vi "Write Duration.vi"(8 "error in (no error)":errorcluster, 10 "Duration":u32 caption="ms" step=1 format="%.0g", 11 "TimedDirector in":refnum<class "TimedDirector.lvclass">) -> (0 "error out":errorcluster, 3 "TimedDirector out":refnum<class "TimedDirector.lvclass">)   [LabVIEW 2023, in "HAF.lvlib" / "TimedDirector.lvclass"]
uses:
  TimedDirector.lvclass
  TimedDirector.lvclass/TimedDirector.ctl
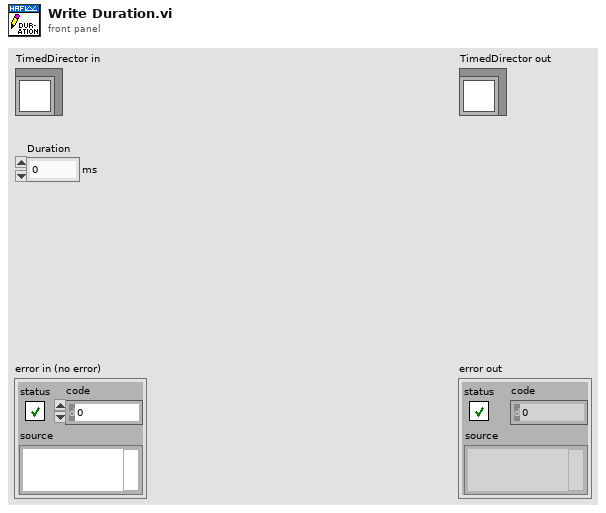
[diagram p1: front panel]
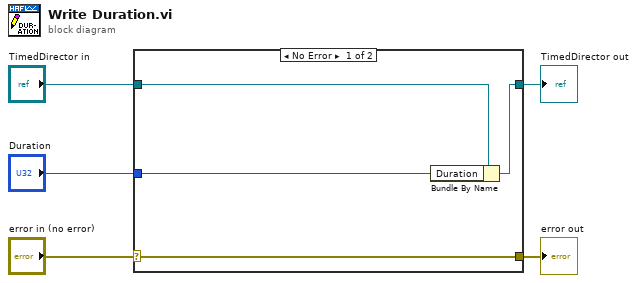
[diagram p0: block diagram]
diagram:
  n1 = case shown="No Error" "error in (no error)" {
    selector: "error in (no error)" -> [w9 w10]
    tunnel: [w9 w10] -> w4
    tunnel: [w7 w11] -> w2
    tunnel: "TimedDirector in" -> [w8 w11]
    tunnel: "Duration" -> [w6 _]
    frame No Error {
      n2 = Bundle By Name(cluster=w8, "Duration"=w6) -> (w7:refnum<class "TimedDirector.lvclass">)
    }
    frame Error {
    }
  }
  "error out" <- w4
  "TimedDirector out" <- w2
